vi "实验3-2.vi"() -> ()   [LabVIEW 2018]
panel:
  out "平均值":dbl
  out "最大值":dbl
  out "最小值":dbl=1.0
  in  "?":bool
  out "?":cluster{dbl, dbl}(graph)
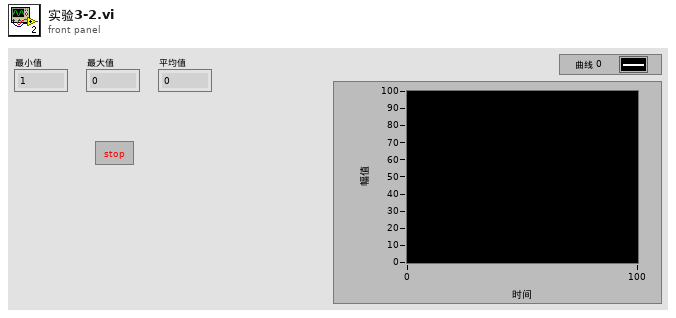
[diagram p1: front panel]
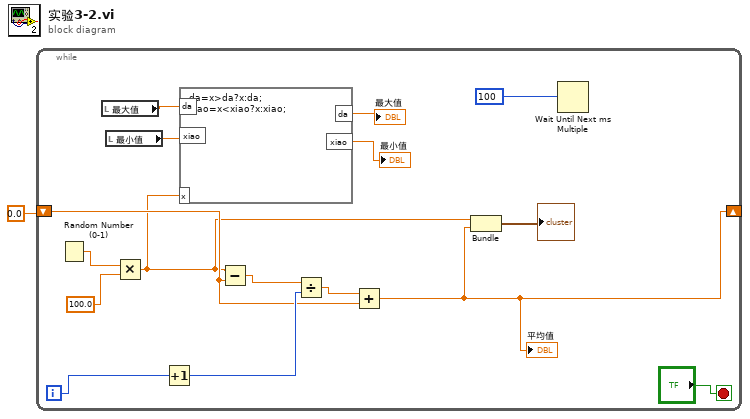
[diagram p0: block diagram]
diagram:
  n1 = while {
    shift-right: [w5] -> _
    shift-left: 0.0 -> [w7]
    i -> [w10]
    stop <- "?" stop-if-true
    n2 = Random Number (0-1)() -> (number: 0 to 1=w13:dbl)
    n3 = local read "最大值"() -> (w15:dbl)
    n4 = local read "最小值"() -> (w14:dbl)
    n5 = Multiply(x=w13, y=100.0) -> (x*y=w6:dbl)
    n6 = Increment(x=w10) -> (x+1=w9:i32)
    n7 = formula code="da=x>da?x:da;\nxiao=x<xiao?x:xiao;"("da"=w15, "xiao"=w14, "x"=w6) -> ("da"=→"最大值":dbl, "xiao"=→"最小值":dbl)
    n8 = Subtract(x=w6, y=w7) -> (x-y=w11:dbl)
    n9 = Divide(x=w11, y=w9) -> (x/y=w8:dbl)
    n10 = Add(x=w8, y=w7) -> (x+y=w5:dbl)
    "平均值" <- w5
    n11 = Bundle(w6, w5) -> (→"?":cluster{dbl, dbl})  [unwired: 1 in]
    n12 = Wait Until Next ms Multiple(millisecond multiple=100) -> ()  [unwired: 1 out]
  }
